vi "Meas_Frequency.vi"(0 "Semiconductor Module Context":T5, 1 "Scope_Master_Controls":T1={"Scope_Vertical_Settings"={"Vertical Range (V)"=5.0, "Vertical Coupling"=1, "Input Impedance"=0}, "Scope_Horizontal_Settings"={"Min Record Length"=4000, "Min. Sample Rate"=200000000.0}, "Scope_Trigger_Settings"={"Trigger Level (V)"=0.75, "Trigger Slope"=0, "Coupling"=1, "Trigger Modifier"=2}} {"Scope_Trigger_Settings"."Trigger Modifier" items=["None"=1, "Auto Trigger"=2]; "Scope_Trigger_Settings"."Coupling" items=["AC"=0, "DC"=1, "HF Reject"=3, "LF Reject"=4, "AC Plus HF Reject"=1001]; "Scope_Trigger_Settings"."Trigger Slope" items=["Positive", "Negative"]; "Scope_Trigger_Settings"."Trigger Level (V)" format="%.2f"; "Scope_Horizontal_Settings"."Min. Sample Rate" format="%#_6p"; "Scope_Vertical_Settings"."Input Impedance" items=["1 mega ohm"=0, "50 ohms"=2]; "Scope_Vertical_Settings"."Vertical Coupling" items=["AC", "DC", "Ground"]; "Scope_Vertical_Settings"."Vertical Range (V)" format="%_3g"}, 2 "scalar measurement":T6=1016 caption="Measurement" items=["None"=4000, "Frequency"=2, "Average Frequency"=1016, "FFT Frequency"=1008, "Period"=3, "Average Period"=1015, "Rise Time"=0, "Fall Time"=1, "Rising Slew Rate"=1010, "Falling Slew Rate"=1011, "Overshoot"=18, "Preshoot"=19, "Voltage RMS"=4, "Voltage Cycle RMS"=16, "AC Estimate"=1012, "FFT Amplitude"=1009, "Voltage Average"=10, "Voltage Cycle Average"=17, "DC Estimate"=1013, "Voltage Max"=6, "Voltage Min"=7, "Voltage Peak-to-Peak"=5, "Voltage High"=8, "Voltage Low"=9, "Voltage Amplitude"=15, "Voltage Top"=1007, "Voltage Base"=1006, "Voltage Base-to-Top"=1017, "Negative Width"=11, "Positive Width"=12, "Negative Duty Cycle"=13, "Positive Duty Cycle"=14, "Integral"=1005, "Area"=1003, "Cycle Area"=1004, "Time Delay"=1014, "Phase Delay"=1018, "Low Ref Volts"=1000, "Mid Ref Volts"=1001, "High Ref Volts"=1002, "Volt. Hist. Mean"=2000, "Volt. Hist. Stdev"=2001, "Volt. Hist. Median"=2003, "Volt. Hist. Mode"=2010, "Volt. Hist. Max"=2005, "Volt. Hist. Min"=2006, "Volt. Hist. Peak-to-Peak"=2002, "Volt. Hist. Mean + Stdev"=2007, "Volt. Hist. Mean + 2 Stdev"=2008, "Volt. Hist. Mean + 3 Stdev"=2009, "Volt. Hist. Hits"=2004, "Volt. Hist. New Hits"=2011, "Time Hist. Mean"=3000, "Time Hist. Stdev"=3001, "Time Hist. Median"=3003, "Time Hist. Mode"=3010, "Time Hist. Max"=3005, "Time Hist. Min"=3006, "Time Hist. Peak-to-Peak"=3002, "Time Hist. Mean + Stdev"=3007, "Time Hist. Mean + 2 Stdev"=3008, "Time Hist. Mean + 3 Stdev"=3009, "Time Hist. Hits"=3004, "Time Hist. New Hits"=3011], 5 "Pins":string[](array[string]), 7 "Locals_Trim_Value":dbl, 11 "Error In":errorcluster) -> (4 "SOI_CLK_Freq_Mhz":dbl, 15 "Error Out":errorcluster)   [LabVIEW 2013]
uses:
  <instrlib>/niScope/Controls/niScope scalar measurement.ctl
  <vilib>/NI_TestStand_SemiconductorModule/NI_TestStand_Semiconductor_Module.lvlibp/PinMap/General/SemiconductorModuleContext.ctl
  Controls/Scope_Master_Controls.ctl
  Controls/Scope_Vertical_Settings.ctl
  Controls/Scope_Horizontal_Settings.ctl
  Controls/Scope_Trigger_Settings.ctl
  <instrlib>/niScope/Configure/Trigger/niScope Configure Trigger Edge.vi
  <instrlib>/niScope/Acquire/niScope Read Cluster.vi
  <instrlib>/niScope/Measurements/niScope Fetch Measurement.vi
  <vilib>/NI_TestStand_SemiconductorModule/NI_TestStand_Semiconductor_Module.lvlibp
panel:
  out "Measured_Freq_Mhz":dbl
  out "Waveform From Scope":T7(graph) caption="Waveform from Scope"
  # "Triggering"
  # "Horizontal"
  # "Vertical"
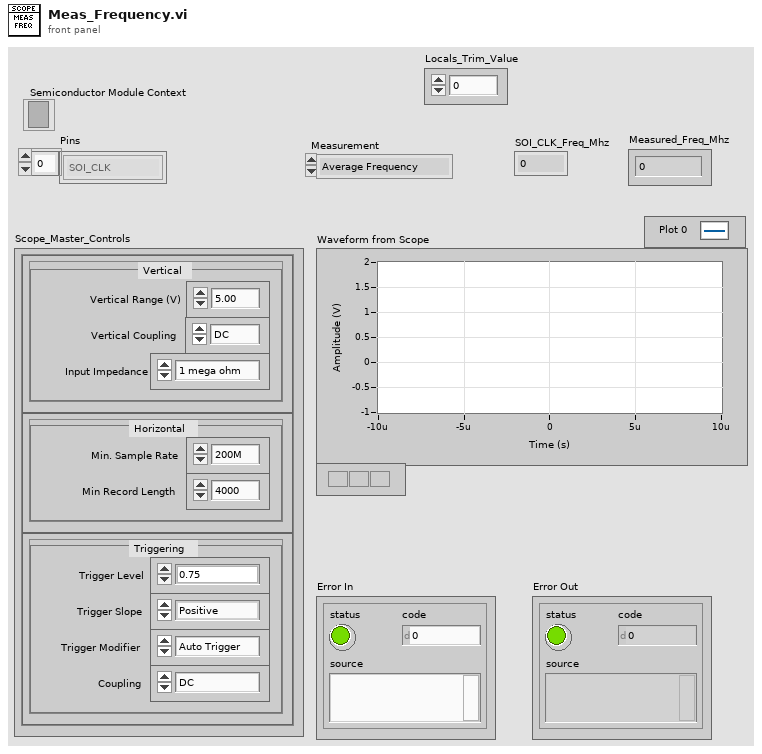
[diagram p1: front panel]
types:
  T1 = typedef "Scope_Master_Controls.ctl" = cluster{"Scope_Vertical_Settings":T2, "Scope_Horizontal_Settings":T3, "Scope_Trigger_Settings":T4}
  T2 = typedef "Scope_Vertical_Settings.ctl" = cluster{"Vertical Range (V)":dbl, "Vertical Coupling":i32, "Input Impedance":u32}
  T3 = typedef "Scope_Horizontal_Settings.ctl" = cluster{"Min Record Length":i32, "Min. Sample Rate":dbl}
  T4 = typedef "Scope_Trigger_Settings.ctl" = cluster{"Trigger Level (V)":dbl, "Trigger Slope":i32, "Coupling":u16, "Trigger Modifier":i32}
  T5 = typedef "NI_TestStand_Semiconductor_Module.lvlibp/SemiconductorModuleContext.ctl" = refnum<k7>
  T6 = typedef "niScope scalar measurement.ctl" = i32
  T7 = cluster{"relativeInitialX":dbl, "xIncrement":dbl, "wfm":dbl[]}
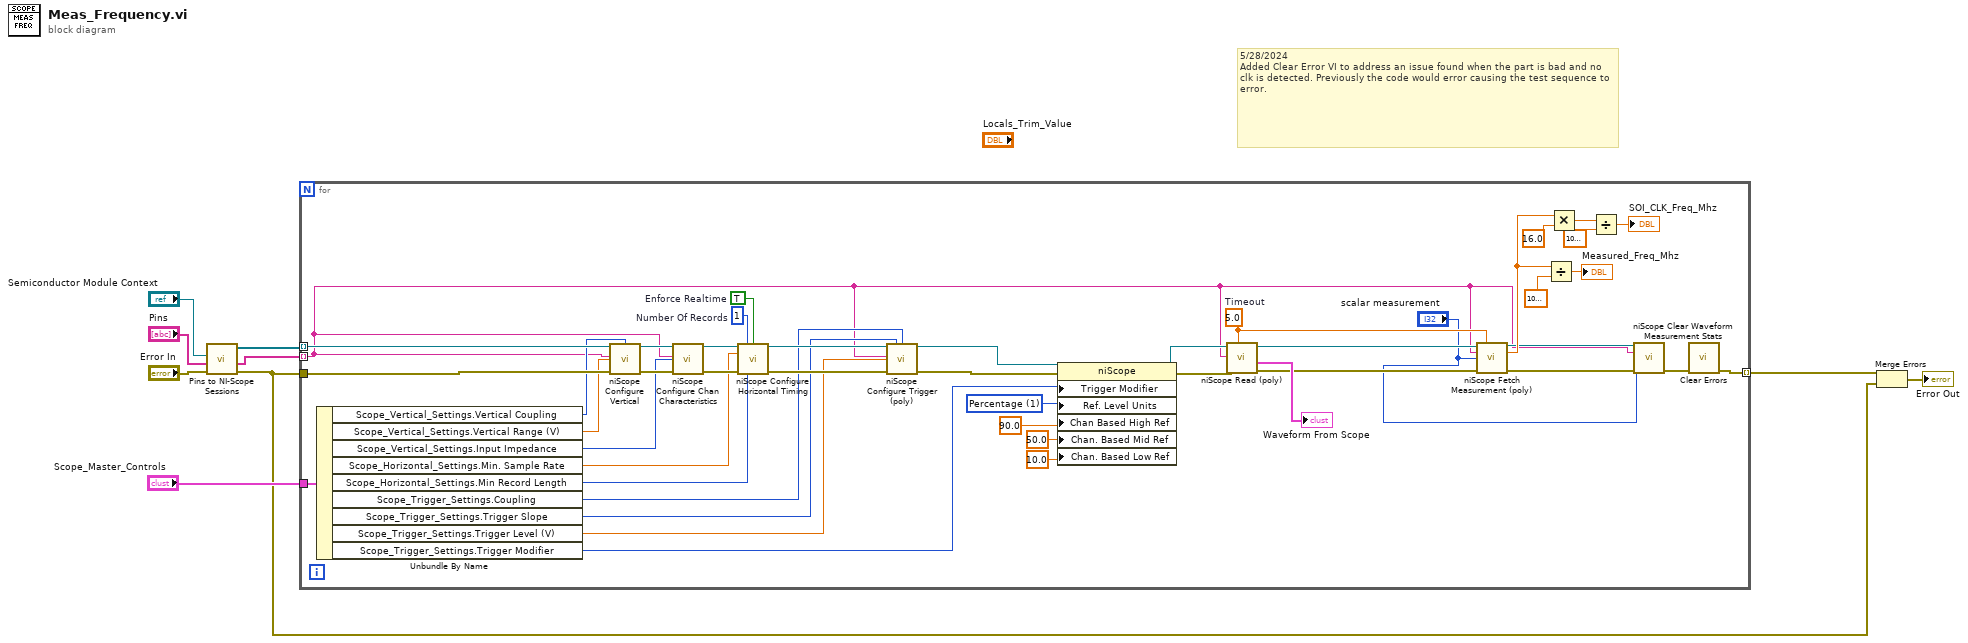
[diagram p0: block diagram]
diagram:
  # "5/28/2024\nAdded Clear Error VI to address an issue found when the part is bad and no clk is detected. Previously the code would error causing the test sequence to error."
  n1 = call "Pins to NI-Scope Sessions.vi"("error in (no error)"="Error In", "Pins"="Pins", "Semiconductor Module Context"="Semiconductor Module Context") -> ("error out"=w3:errorcluster, "Channel Lists"=w6:string[], "Instrument Sessions"=w7:refnum<k15>[])  [unwired: 5 in, 1 out]
  n2 = for {
    tunnel: w7 -> [w38] mode=indexing
    tunnel: w3 -> [w37]
    tunnel: w6 -> [w15] mode=indexing
    tunnel: "Scope_Master_Controls" -> [w36]
    tunnel: [w19] -> w4 mode=indexing
    w13 = 1 items=["Volts", "Percentage"] ("Waveform Measurement:Reference Levels:Units")
    w39 = TRUE  # Enforce Realtime
    w40 = 1  # Number Of Records
    w45 = 5.0  # Timeout
    n3 = Unbundle By Name(w36) -> ("Scope_Vertical_Settings.Vertical Coupling"=w29:i32, "Scope_Vertical_Settings.Vertical Range (V)"=w35:dbl, "Scope_Vertical_Settings.Input Impedance"=w34:u32, "Scope_Horizontal_Settings.Min. Sample Rate"=w33:dbl, "Scope_Horizontal_Settings.Min Record Length"=w32:i32, "Scope_Trigger_Settings.Coupling"=w27:u16, "Scope_Trigger_Settings.Trigger Slope"=w28:i32, "Scope_Trigger_Settings.Trigger Level (V)"=w31:dbl, "Scope_Trigger_Settings.Trigger Modifier"=w30:i32)
    n4 = call <instrlib>:"niScope Configure Vertical.vi"("instrument handle"=w38, "vertical coupling"=w29, "channels"=w15, "vertical range"=w35, "error in"=w37) -> ("instrument handle out"=w43:refnum<k15>, "error out"=w44:errorcluster)  [unwired: 9 in]
    n5 = call <instrlib>:"niScope Configure Chan Characteristics.vi"("instrument handle"=w43, "channels"=w15, "input impedance"=w34, "error in"=w44) -> ("instrument handle out"=w42:refnum<k15>, "error out"=w41:errorcluster)  [unwired: 10 in]
    n6 = call <instrlib>:"niScope Configure Horizontal Timing.vi"("instrument handle"=w42, "number of records"=w40, "enforce realtime"=w39, "min sample rate"=w33, "error in"=w41, "min record length"=w32) -> ("instrument handle out"=w52:refnum<k15>, "error out"=w53:errorcluster)  [unwired: 8 in]
    n7 = call-poly <instrlib>:"niScope Configure Trigger (poly).vi"("instrument handle"=w52, "trigger slope"=w28, "trigger coupling"=w27, "trigger source"=w15, "trigger level"=w31, "error in"=w53) -> ("instrument handle out"=w49:refnum<k15>, "error out"=w48:errorcluster)  [unwired: 8 in]
    n8 = property class="niScope"(reference=w49, error in=w48, "Trigger Modifier"=w30, "Ref. Level Units"=w13, "Chan Based High Ref"=90.0 ("Waveform Measurement:Reference Levels:Channel Based High Ref Level"), "Chan. Based Mid Ref"=50.0 ("Waveform Measurement:Reference Levels:Channel Based Mid Ref Level"), "Chan. Based Low Ref"=10.0 ("Waveform Measurement:Reference Levels:Channel Based Low Ref Level")) -> (reference out=w46:refnum<k15>, error out=w47:errorcluster)
    n9 = call-poly <instrlib>:"niScope Read (poly).vi"("timeout"=w45, "error in"=w47, "channels"=w15, "instrument handle"=w46) -> ("error out"=w50:errorcluster, "waveform"=→"Waveform From Scope":T7, "instrument handle out"=w51:refnum<k15>)  [unwired: 4 in, 1 out]
    n10 = call-poly <instrlib>:"niScope Fetch Measurement (poly).vi"("instrument handle"=w51, "timeout"=w45, "channels"=w15, "scalar measurement"="scalar measurement", "error in"=w50) -> ("instrument handle out"=w16:refnum<k15>, "result"=w23:dbl, "error out"=w17:errorcluster)  [unwired: 8 in]
    n11 = Divide(x=w23, y=1000000.0) -> (x/y=→"Measured_Freq_Mhz":dbl)
    n12 = Multiply(x=w23, y=16.0) -> (x*y=w22:dbl)
    n13 = Divide(x=w22, y=1000000.0) -> (x/y=→"SOI_CLK_Freq_Mhz":dbl)
    n14 = call <instrlib>:"niScope Clear Waveform Measurement Stats.vi"("instrument handle"=w16, "channels"=w15, "clearable measurement"="scalar measurement", "error in"=w17) -> ("error out"=w18:errorcluster)  [unwired: 10 in, 1 out]
    n15 = call <vilib>:"Clear Errors.vi"("error in (no error)"=w18) -> ("error out"=w19:errorcluster)  [unwired: 6 in]
  }
  n16 = Merge Errors(w4, w3) -> (→"Error Out":errorcluster)
